vi "launch_auto_test.vi"(8 "error in (no error)":errorcluster, 9 "user_event_out":T1, 10 "modbusData":refnum<notifier>, 11 "Cluster":T2) -> (0 "error out":errorcluster)   [LabVIEW 2019]
uses:
  core_dataRefCluster.ctl
  core_dataRef.ctl
  core_dataCluster.ctl
  instrument/instr_dataCluster.ctl
  gui/test_result_user_event1.ctl
  gui/test_results 1.ctl
  instrument/Instrument.lvclass
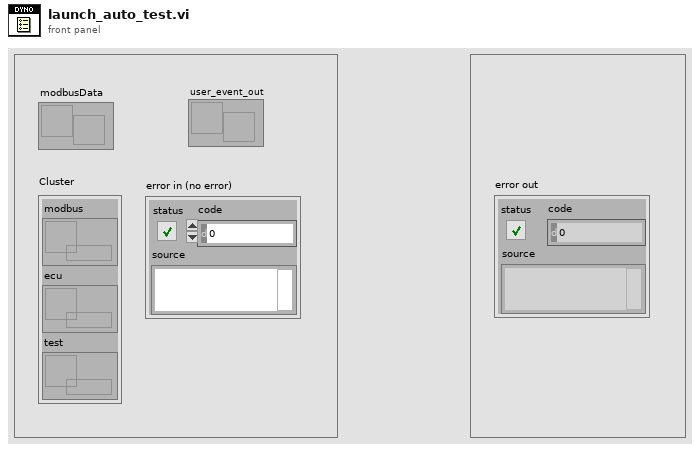
[diagram p1: front panel]
types:
  T1 = typedef "test_result_user_event1.ctl" = refnum<user-event>
  T2 = typedef "core_dataRefCluster.ctl" = cluster{"modbus":T3, "ecu":T3, "test":T3}
  T3 = typedef "core_dataRef.ctl" = refnum<queue>
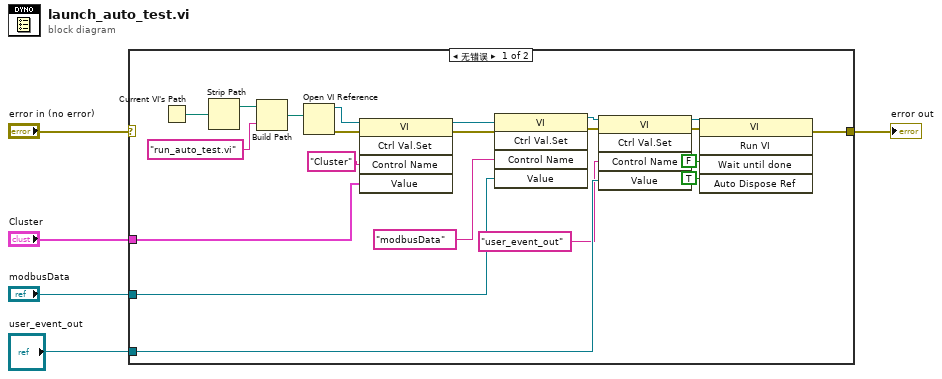
[diagram p0: block diagram]
diagram:
  n1 = case shown="无错误" "error in (no error)" {
    selector: "error in (no error)" -> [_ w27]
    tunnel: "Cluster" -> [w24 _]
    tunnel: "modbusData" -> [w23 _]
    tunnel: [w12 w27] -> w3
    tunnel: "user_event_out" -> [w7 _]
    frame No Error {
      n2 = Current VI's Path() -> (path=w20:path)
      n3 = Strip Path(path=w20) -> (stripped path=w19:path)  [unwired: 1 out]
      n4 = Build Path(base path=w19, name or relative path="run_auto_test.vi") -> (appended path=w17:path)
      n5 = Open VI Reference(vi path=w17) -> (vi reference=w26:refnum<vi>, error out=w21:errorcluster)  [unwired: 5 in]
      n6 = invoke class="VI" method="Ctrl Val.Set"(reference=w26, error in=w21, "Control Name"="Cluster", "Value"=w24) -> (reference out=w25:refnum<vi>, error out=w22:errorcluster)  [unwired: 1 in, 3 out]
      n7 = invoke class="VI" method="Ctrl Val.Set"(reference=w25, error in=w22, "Control Name"="modbusData", "Value"=w23) -> (reference out=w9:refnum<vi>, error out=w8:errorcluster)  [unwired: 1 in, 3 out]
      n8 = invoke class="VI" method="Ctrl Val.Set"(reference=w9, error in=w8, "Control Name"="user_event_out", "Value"=w7) -> (reference out=w11:refnum<vi>, error out=w10:errorcluster)  [unwired: 1 in, 3 out]
      n9 = invoke class="VI" method="Run VI"(reference=w11, error in=w10, "Wait until done"=FALSE ("Wait Until Done"), "Auto Dispose Ref"=TRUE ("Auto Dispose Reference")) -> (error out=w12:errorcluster)  [unwired: 1 in, 4 out]
    }
    frame Error {
    }
  }
  "error out" <- w3
